vi "Create.vi"(6 "LabPack Shared Library":path=path "", 8 "Error In":errorcluster) -> (0 "Error Out":errorcluster, 3 "Reader":refnum<class "Reader.lvclass">)   [LabVIEW 2017, in "LabPack.lvlib" / "Reader.lvclass"]
doc: "Creates a default object of the Reader class for reading and decoding MessagePack data."
uses:
  Reader.lvclass
  Reader.lvclass/Reader.ctl
  Status/Read Status.vi
  Status/Read Status Message.vi
  Status/Read Is Error.vi
  Utility/Status Code.vi
  <vilib>/Utility/error.llb/Error Cluster From Error Code.vi
  LabPack.lvlib
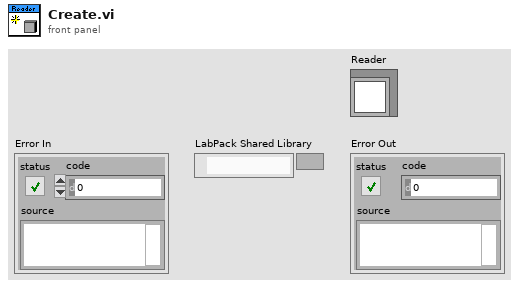
[diagram p1: front panel]
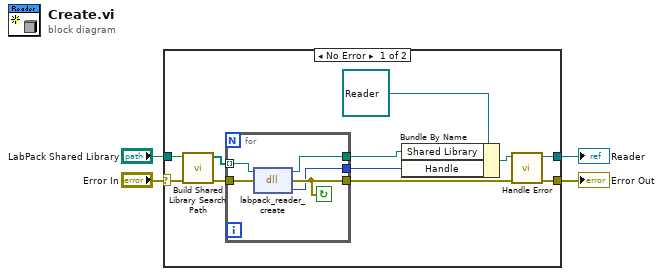
[diagram p0: block diagram]
diagram:
  n1 = case shown="No Error" "Error In" {
    selector: "Error In" -> [w14 w21]
    tunnel: "LabPack Shared Library" -> [w15 _]
    tunnel: [w7 _] -> w2
    tunnel: [w5 w21] -> w1
    frame No Error {
      n2 = call "Build Shared Library Search Path.vi"("Error In"=w14, "LabPack Shared Library"=w15) -> ("Error Out"=w12:errorcluster, "Search Path"=w13:path[])  [unwired: 8 in]
      n3 = for {
        tunnel: w13 -> [w18] mode=indexing
        tunnel: w12 -> [w20]
        tunnel: [w19] -> w6
        tunnel: [w17] -> w10
        tunnel: [w16] -> w9
        stop <- w19 continue-if-true
        n4 = dll-call lib="D:/Users/cfield/Code/MessagePack/LabPack/LabVIEW/trunk/src/LabPack/Private/labpack-x64.dll" fn="labpack_reader_create"(path in=w18, error in=w20) -> (path out=w17:path, error out=w19:errorcluster, "return type"=w16:u64)  [unwired: 1 in]
      }
      n5 = Bundle By Name(cluster=refnum<class "Reader.lvclass"> refnum ("LabPack.lvlib:Reader.lvclass"), "Shared Library"=w10, "Handle"=w9) -> (w8:refnum<class "Reader.lvclass">)
      n6 = call "Handle Error.vi"("Error In"=w6, "Reader In"=w8) -> ("Error Out"=w5:errorcluster, "Reader Out"=w7:refnum<class "Reader.lvclass">)  [unwired: 8 in]
    }
    frame Error {
    }
  }
  "Reader" <- w2
  "Error Out" <- w1
